vi "Unindent All String.vi"(8 "error in (no error)":errorcluster, 9 "Width (4)":u32=4, 10 "Count (1)":u32=1, 11 "String":string) -> (0 "error out":errorcluster, 3 "String out":string)   [LabVIEW 2015, in "YAML Parser.lvclass"]
uses:
  YAML Parser.lvclass
panel:
  out "number of replacements":i32
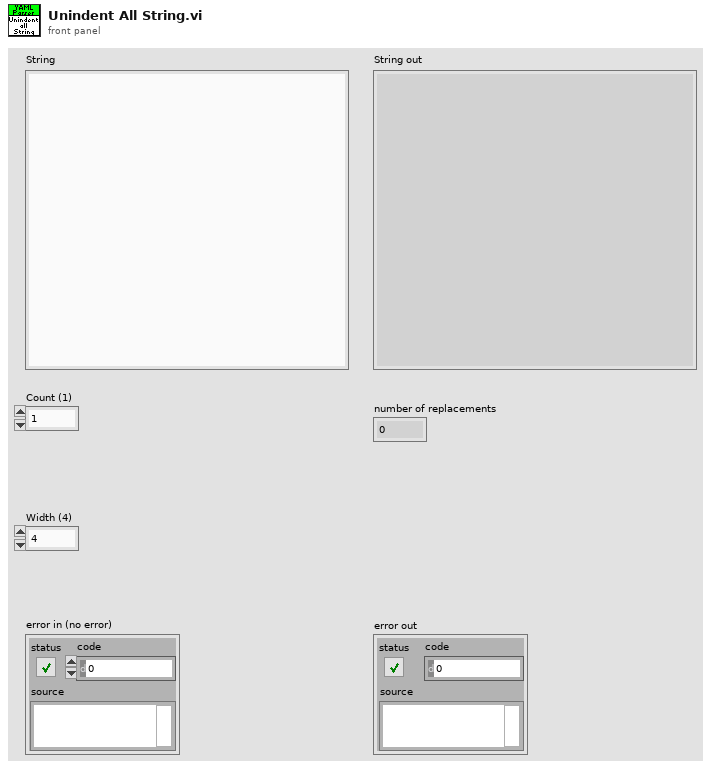
[diagram p1: front panel]
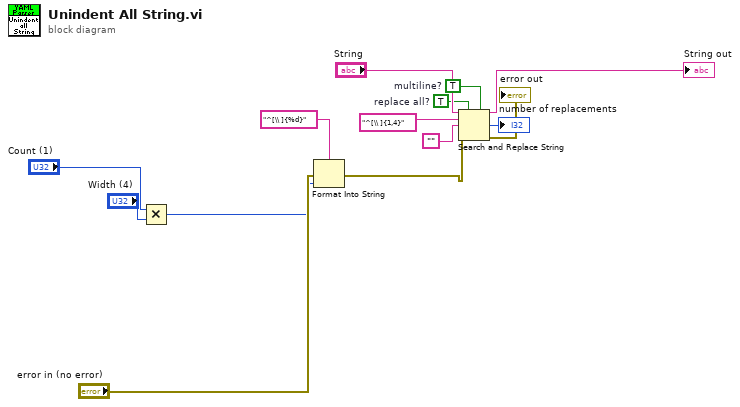
[diagram p0: block diagram]
diagram:
  w11 = TRUE  # replace all?
  w12 = TRUE  # multiline?
  n1 = Multiply(x="Count (1)", y="Width (4)") -> (x*y=w2:u32)
  n2 = Format Into String(format string="^[\\ ]{%d}" ("search string"), error in="error in (no error)", w2) -> (error out=w4:errorcluster)  [unwired: 1 in, 1 out]
  n3 = Search and Replace String(replace all?=w11, multiline?=w12, input string="String", search string="^[\\ ]{1,4}", replace string="", error in=w4) -> (result string=→"String out":string, number of replacements=→"number of replacements":i32, error out=→"error out":errorcluster)  [unwired: 2 in, 1 out]
